vi "FF_compute2.vi"(0 "InitialCenter":dbl[](array[numeric]), 1 "CenPt":dbl[](array[numeric]), 2 "FrameNum":dbl, 7 "xyz_o":dbl[][](array[numeric]), 11 "New Center":dbl[](array[numeric]), 12 "Use FF":bool) -> (4 "P'":dbl[](array[numeric]), 5 "TraFF":dbl[](array[numeric]), 6 "curr Point":dbl[](array[numeric]), 8 "ForceAll":dbl[](array[numeric]), 10 "Closest Pt":dbl[](array[numeric]), 14 "InitalCenterOut":dbl[](array[numeric]), 15 "DesiredFM_FF":dbl[](array[numeric]))   [LabVIEW 2017]
uses:
  typeDef/AnkleTraj.ctl
  <vilib>/Analysis/_algsub.llb/Real Vector Norm.vi
  <vilib>/Analysis/baseanly.llb/Real Dot Product.vi
  <vilib>/Analysis/BLAS.llb/idamin - Min Element Index (DBL).vi
  <vilib>/Analysis/NI_AALBase.lvlib
  <vilib>/Analysis/NI_AALPro.lvlib
  <vilib>/Analysis/NI_AALBLAS.lvlib
panel:
  out "subarray 2":dbl[](array[numeric])
  out "subarray":dbl[](array[numeric])
  in  "Fz":dbl=20.0
  out "Desired FM_FF":dbl[](array[numeric])
  out "sqrt(x)":dbl
  out "P1 full size":i32[](array[numeric])
  out "P2 full":dbl[][](array[numeric])
  out "P1 full":dbl[][](array[numeric])
  out "CheckPlus":dbl[][](array[numeric])
  in  "AnkleTraj":T1
  out "OrderOfClosePt":i32
  in  "MxMyMz":dbl[](array[numeric])=[5.0, 5.0, 5.0, 4.0, 4.0, 4.0]
  in  "Enum":enum16{"Linear", "Bell"}(ring)=enum."Bell"
  out "ForceComp":dbl[](array[numeric])
  out "n_dir":dbl[](array[numeric])
  out "d_min":dbl
  out "ForceXYZ":dbl[](array[numeric])
  out "NormalVectorToClosestPt":dbl[](array[numeric])
  out "DistanceToClosestPt":dbl
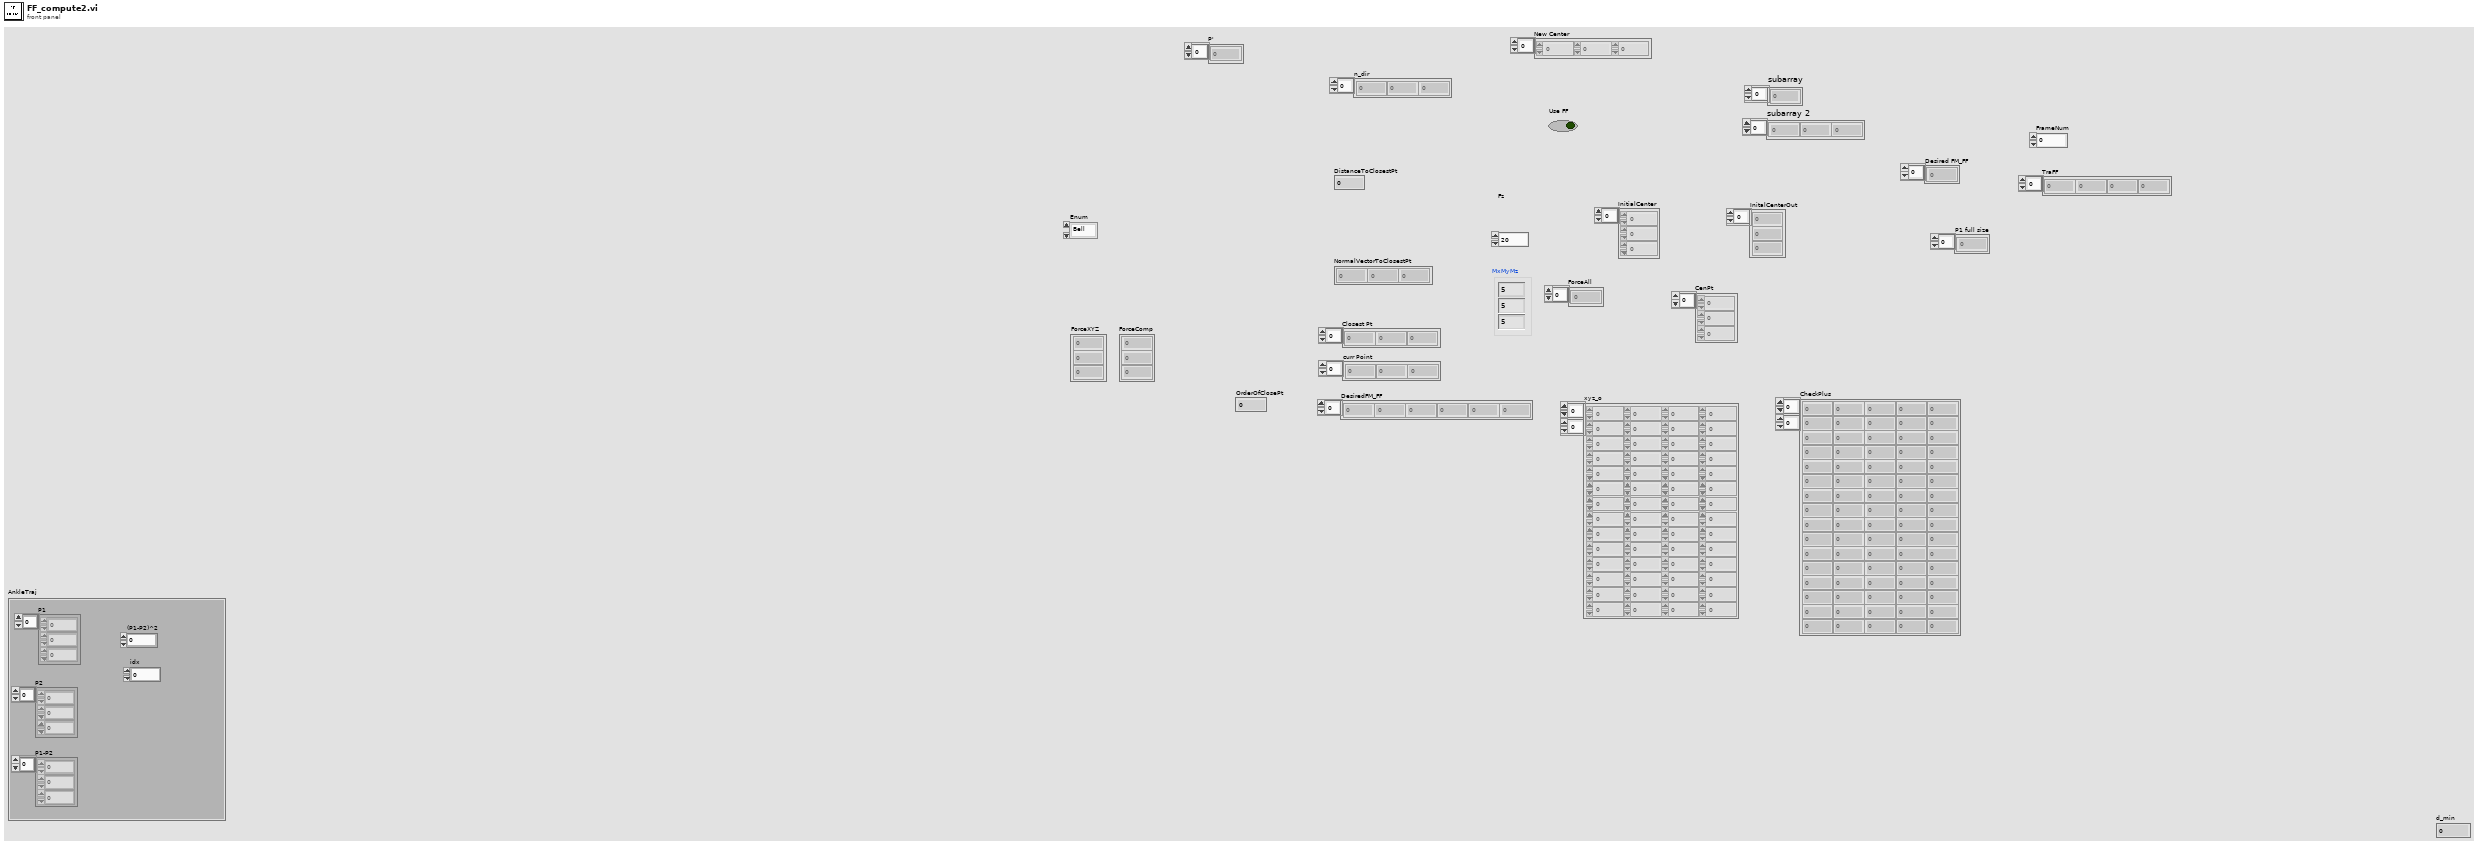
[diagram p1: front panel]
types:
  T1 = typedef "AnkleTraj.ctl" = cluster{"P1":dbl[], "P2":dbl[], "P1-P2":dbl[], "(P1-P2)^2":dbl, "idx":i32}
  T2 = cluster{"Kn":dbl, "Kt":dbl, "Kd_n":dbl, "Dn":dbl, "Dt":dbl, "Kd_t":dbl}
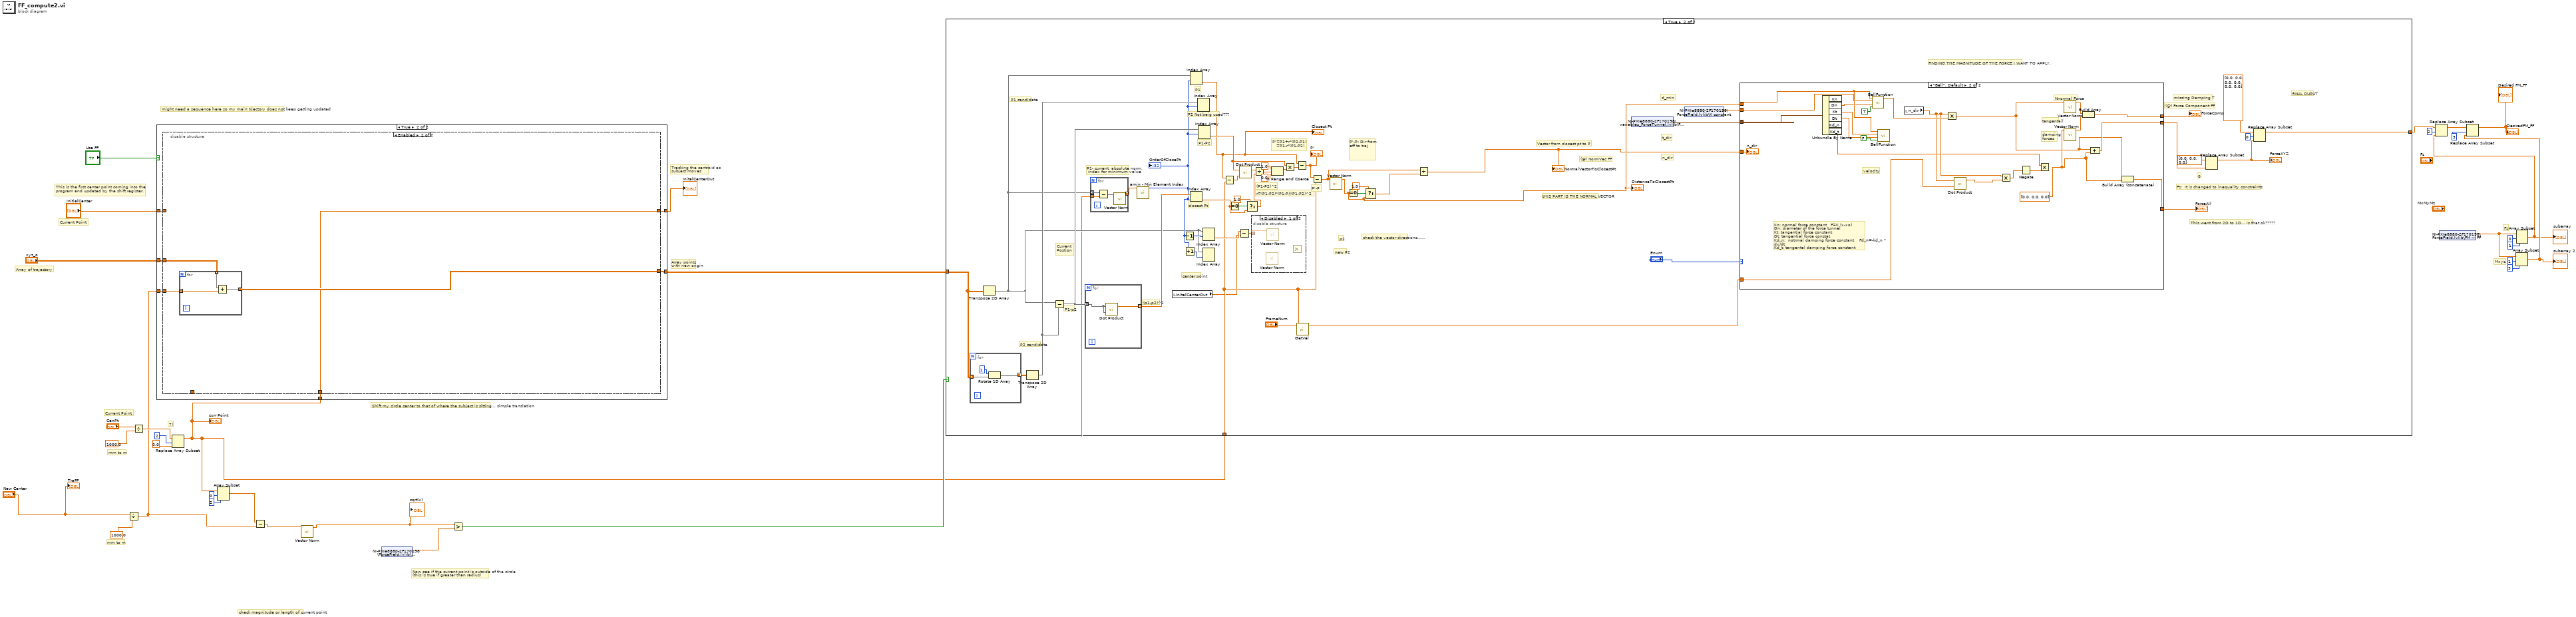
[diagram p0: block diagram]
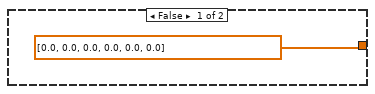
[diagram p2: hidden frame]
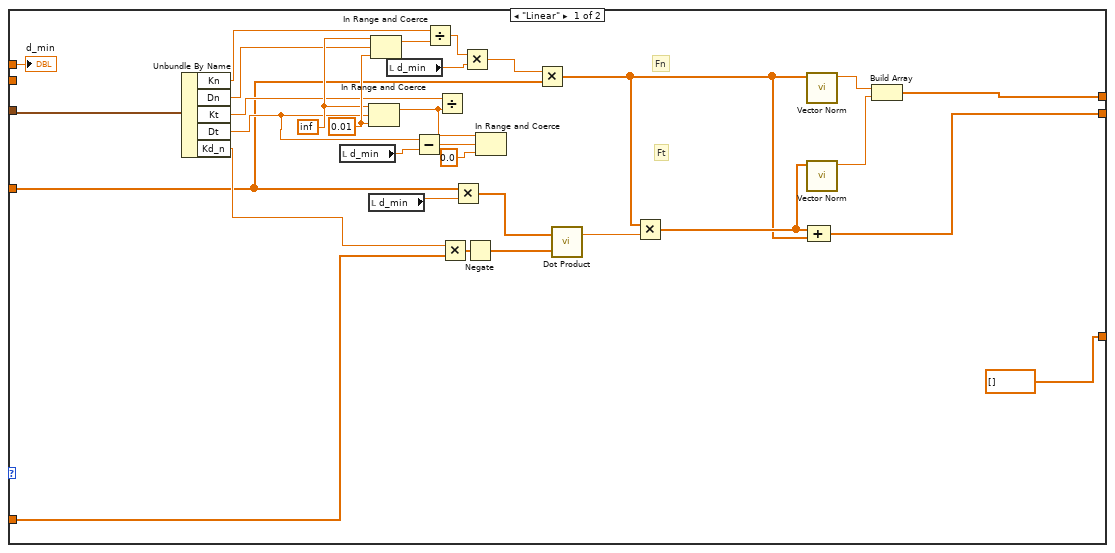
[diagram p4: hidden frame]
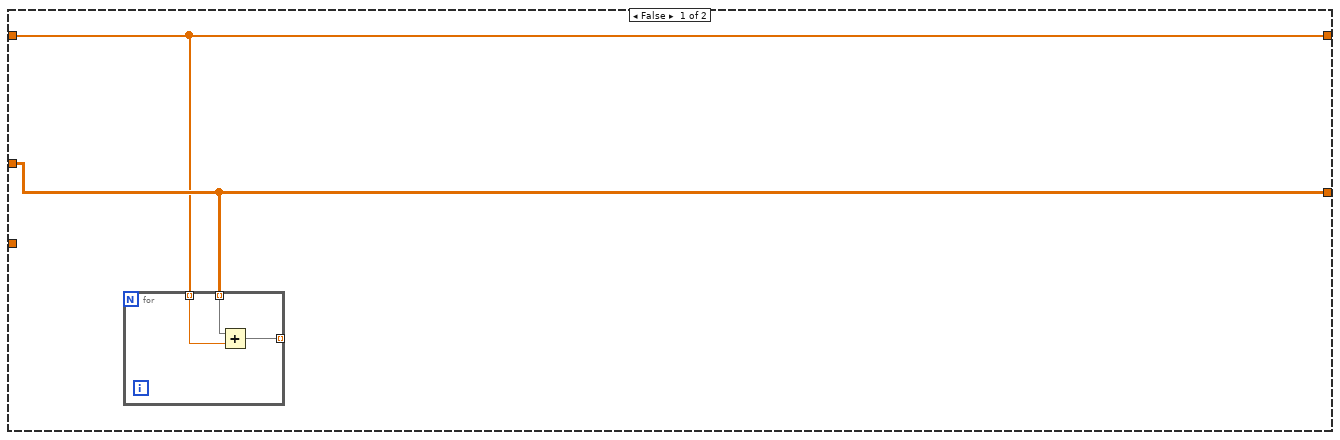
[diagram p5: hidden frame]
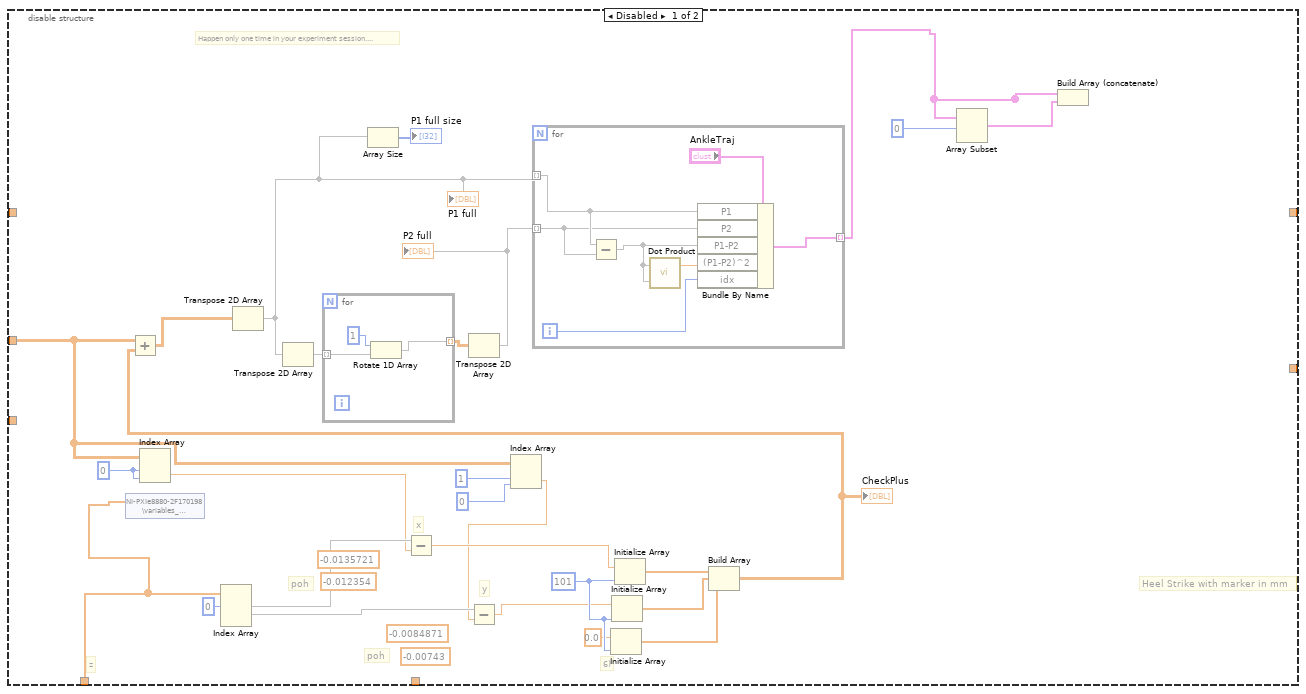
[diagram p6: hidden frame]
diagram:
  # "Current Point"
  # "Current Point"
  # "Fz"
  # "Mxyz"
  # "This is the first center point coming into the\nprogram and updated by the shift register."
  # "Now see if the current point is outside of the circle\n(this is true if greater than radius)"
  # "check magnitude or length of current point"
  # "mm to m"
  # "Tracking the centroid as \nsubject moves"
  # "might need a sequence here so my main trjectory does not keep getting updated"
  # "Array points \nwith new origin"
  # "Shift my circle center to that of where the subject is sitting... simple translation"
  # "mm to m"
  # "Array of trajectory"
  # "7)"
  n1 = Divide(x="New Center", y=1000.0) -> (x/y=w16:dbl[])
  n2 = Divide(x="CenPt", y=1000.0) -> (x/y=w28:dbl[])
  n3 = Replace Array Subset(array=w28, new element=0.0 ("new element/subarray"), index=2) -> (w15:dbl[])
  "curr Point" <- w15
  n4 = case shown="True" "Use FF" {
    tunnel: "xyz_o" -> [w35 w44]
    tunnel: [w35 w43] -> w26
    tunnel: "InitialCenter" -> [w34 w42]
    tunnel: [w34 w41] -> w24
    tunnel: w15 -> [_ w40]
    tunnel: w16 -> [_ w39]
    frame False {
      n5 = for {
        tunnel: w35 -> [w38] mode=indexing
        tunnel: [w37] -> _ mode=indexing
        tunnel: w34 -> [w36] mode=indexing
        n6 = Add(x=w38, y=w36) -> (x+y=w37:dbl[])
      }
    }
    frame True {
      n7 = disable-structure shown="Enabled" {
        disable-tunnel: _ -> [w51 _]
        disable-tunnel: w44 -> [w48 w86]
        disable-tunnel: [_ w85] -> w43
        disable-tunnel: w42 -> [_ _]
        disable-tunnel: [_ w84] -> w41
        disable-tunnel: w40 -> [_ w84]
        disable-tunnel: w39 -> [_ w83]
        frame Disabled {
          w50 = 0 ("index (row)")
          (unwired) -0.00743 ("x")
          (unwired) -0.012354 ("x")
          (unwired) -0.0084871 ("x")
          (unwired) -0.0135721 ("x")
          w65 = 101 ("dimension size")
          # "Happen only one time in your experiment session...."
          # "poh"
          # "poh"
          # "z"
          # "y"
          # "x"
          # "6)"
          # "Heel Strike with marker in mm"
          n8 = shared-variable "NI-PXIe8880-2F170198\\variables_ForceTunnel.lvlib\\Traj FF"(w51) -> ()  [unwired: 1 in, 1 out]
          n9 = Index Array(array=w48, index (row)=w50, index (col)=w50) -> (element=w49:dbl)
          n10 = Index Array(array=w51, index #1=0 ("index")) -> (element #1=w57, element #2=w59)  [unwired: 2 in, 1 out]
          n11 = Subtract(x=w57, y=w49) -> (x-y=w56:dbl)
          n12 = Index Array(array=w48, index (row)=1 ("disabled index (col)"), index (col)=0 ("index (row)")) -> (element=w47:dbl)
          n13 = Subtract(x=w59, y=w47) -> (x-y=w58:dbl)
          n14 = Initialize Array(0.0 ("element"), w65) -> (w63:dbl[])
          n15 = Initialize Array(w58, w65) -> (w64:dbl[])
          n16 = Initialize Array(w56, w65) -> (w55:dbl[])
          n17 = Build Array(w55, w64, w63) -> (w62:dbl[][])
          "CheckPlus" <- w62
          n18 = Add(x=w48, y=w62) -> (x+y=w61:dbl[][])
          n19 = Transpose 2D Array(2D array=w61) -> (transposed array=w54:dbl[][])
          "P1 full" <- w54
          n20 = Transpose 2D Array(2D array=w54) -> (transposed array=w69:dbl[][])
          n21 = for {
            tunnel: w69 -> [w82] mode=indexing
            tunnel: [w81] -> w68 mode=indexing
            n22 = Rotate 1D Array(1:w82, 2:1 ("n")) -> (0:w81:dbl[])
          }
          n23 = Array Size(array=w54) -> (size(s)=→"P1 full size":i32[])
          n24 = Transpose 2D Array(2D array=w68) -> (transposed array=w52:dbl[][])
          "P2 full" <- w52
          n25 = for {
            tunnel: w54 -> [w78] mode=indexing
            tunnel: w52 -> [w77] mode=indexing
            tunnel: [w74] -> w67 mode=indexing
            i -> [w73]
            n26 = Subtract(x=w78, y=w77) -> (x-y=w75:dbl[])
            n27 = call-poly <vilib>:"Dot Product.vi"("Y Vector"=w75, "X Vector"=w75) -> ("X * Y"=w76:dbl)  [unwired: 1 out]
            n28 = Bundle By Name(cluster="AnkleTraj", "P1"=w78, "P2"=w77, "P1-P2"=w75, "(P1-P2)^2"=w76, "idx"=w73) -> (w74:T1)
          }
          n29 = Array Subset(array=w67, index=0) -> (w72:T1[])  [unwired: 1 in]
          n30 = Build Array (concatenate)(w67, w72) -> (w71:T1[])
        }
        frame Enabled {
          n31 = for {
            tunnel: w86 -> [w89] mode=indexing
            tunnel: [w88] -> w85 mode=indexing
            tunnel: w83 -> [w87] mode=indexing
            n32 = Add(x=w89, y=w87) -> (x+y=w88:dbl[])
          }
        }
      }
    }
  }
  "InitalCenterOut" <- w24
  n33 = Array Subset(array=w15, index=0, length=2) -> (w12:dbl[])
  n34 = Subtract(x=w12, y=w16) -> (x-y=w11:dbl[])
  n35 = call-poly <vilib>:"Vector Norm.vi"("Input Vector"=w11) -> ("norm"=w10:dbl)  [unwired: 9 in, 1 out]
  "sqrt(x)" <- w10
  n36 = shared-variable "NI-PXIe8880-2F170198\\ForceField.lvlib\\Radius"() -> (w1:dbl)  [unwired: 1 in, 1 out]
  n37 = Greater?(x=w10, y=w1) -> (0:w22:bool)
  n38 = case shown="True" w22 {
    tunnel: [dbl[] [0.0, 0.0, 0.0, 0.0, 0.0, 0.0] w92] -> w19
    tunnel: w26 -> [_ w96]
    tunnel: w15 -> [_ w94]
    frame False {
    }
    frame True {
      # "P2 Not beig used???"
      # "This went from 2D to 1D... is that ok?????"
      # "P1- current, absolute norm,\n index for minimum value"
      # "check the vector directions......"
      # "p1"
      # "new P2"
      # "center point"
      # "(p1-p2)^2"
      # "P1-p2"
      # "P1 candidate"
      # "P2 candidate"
      # "fINAL OUPUT"
      # "tHIS PART IS THE NORMAL VECTOR"
      # "FINDING THE MAGNITUDE OF THE FORCE I WANT TO APPLY."
      # "missing Damping T"
      # "0"
      # "Fz:  It is changed to inequality constraints"
      # "(@) Force Component FF"
      # "(@) NormVec FF"
      # "(P1-P2)^2"
      # "closest Pt"
      # "P1-P2"
      # "P1"
      # "P'-P"
      # "P'-P: Dir from eff to traj"
      # "r=(P1-P2)*(P1-P)/(P1-P2)^2"
      # "P'=P1+r*(P2-P1)\n   =P1-r*(P1-P2)"
      # "Current \nPostion"
      # "t_dir"
      # "n_dir"
      # "d_min"
      # "Vector from closest pt to P"
      n39 = for {
        tunnel: w96 -> [w147] mode=indexing
        tunnel: [w146] -> w107 mode=indexing
        n40 = Rotate 1D Array(1:w147, 2:1 ("n")) -> (0:w146:dbl[])
      }
      n41 = Transpose 2D Array(2D array=w96) -> (transposed array=w95:dbl[][])
      n42 = Transpose 2D Array(2D array=w107) -> (transposed array=w98:dbl[][])
      n43 = Subtract(x=w95, y=w98) -> (x-y=w102:dbl[][])
      n44 = for {
        tunnel: w102 -> [w144] mode=indexing
        tunnel: [w143] -> w101 mode=indexing
        n45 = call-poly <vilib>:"Dot Product.vi"("Y Vector"=w144, "X Vector"=w144) -> ("X * Y"=w143:dbl)  [unwired: 1 out]
      }
      n46 = for {
        tunnel: w94 -> [w142] mode=indexing
        tunnel: w95 -> [w141] mode=indexing
        tunnel: [w139] -> w100 mode=indexing
        n47 = Subtract(x=w141, y=w142) -> (x-y=w140:dbl[])
        n48 = call-poly <vilib>:"Vector Norm.vi"("Input Vector"=w140) -> ("norm"=w139:dbl)  [unwired: 9 in, 1 out]
      }
      n49 = call-poly <vilib>:"amin - Min Element Index.vi"("x"=w100) -> ("idamin"=w97:i32)  [unwired: 9 in, 1 out]
      "OrderOfClosePt" <- w97
      n50 = local read "InitalCenterOut"() -> (w93:dbl[])
      n51 = Decrement(x=w97) -> (x-1=w106:i32)
      n52 = Increment(x=w97) -> (x+1=w105:i32)
      n53 = Index Array(array=w95, index (row)=w97) -> (element=w116:dbl[])  [unwired: 1 in]
      "Closest Pt" <- w116
      n54 = Index Array(array=w101, index=w97) -> (element=w110:dbl)
      n55 = Index Array(array=w98, index (row)=w97) -> ()  [unwired: 1 in, 1 out]
      n56 = Index Array(array=w102, index (row)=w97) -> (element=w123:dbl[])  [unwired: 1 in]
      n57 = Index Array(array=w95, index (row)=w106) -> (element=w104:dbl[])  [unwired: 1 in]
      n58 = Index Array(array=w95, index (row)=w105) -> ()  [unwired: 1 in, 1 out]
      n59 = Subtract(x=w116, y=w94) -> (x-y=w130:dbl[])
      n60 = Equal To 0?(x=w110) -> (x = 0?=w112:bool)
      n61 = Subtract(x=w104, y=w93) -> (x-y=w103:dbl[])
      n62 = call-poly <vilib>:"Dot Product.vi"("Y Vector"=w130, "X Vector"=w123) -> ("X * Y"=w129:dbl)  [unwired: 1 out]
      n63 = Select(t=1.0, s=w112, f=w110) -> (s? t:f=w109:dbl)
      n64 = disable-structure shown="Disabled" {
        disable-tunnel: w103 -> [w138 _]
        frame Disabled {
          n65 = call-poly <vilib>:"Vector Norm.vi"() -> ()  [unwired: 10 in, 2 out]
          n66 = call-poly <vilib>:"Vector Norm.vi"("Input Vector"=w138) -> ()  [unwired: 9 in, 2 out]
          n67 = Greater?() -> ()  [unwired: 2 in, 1 out]
        }
        frame Enabled {
        }
      }
      n68 = Divide(x=w129, y=w109) -> (x/y=w128:dbl)
      n69 = In Range and Coerce(upper limit=1.0, x=w128, lower limit=0.0) -> (coerced(x)=w125:dbl)  [unwired: 1 out]
      n70 = Multiply(x=w123, y=w125) -> (x*y=w124:dbl[])
      n71 = Subtract(x=w116, y=w124) -> (x-y=w121:dbl[])
      "P'" <- w121
      n72 = call "GetVel.vi"("Position"=w94, "FrameNum"="FrameNum") -> ("Velocity"=w118:dbl[])  [unwired: 9 in]
      n73 = Subtract(x=w121, y=w94) -> (x-y=w122:dbl[])
      n74 = call-poly <vilib>:"Vector Norm.vi"("Input Vector"=w122) -> ("norm"=w108:dbl)  [unwired: 9 in, 1 out]
      "DistanceToClosestPt" <- w108
      n75 = Equal To 0?(x=w108) -> (x = 0?=w115:bool)
      n76 = Select(t=1.0, s=w115, f=w108) -> (s? t:f=w113:dbl)
      n77 = Divide(x=w122, y=w113) -> (x/y=w120:dbl[])
      "NormalVectorToClosestPt" <- w120
      n78 = shared-variable "NI-PXIe8880-2F170198\\variables_ForceTunnel.lvlib\\FF Constant"() -> (w117:T2)  [unwired: 1 in, 1 out]
      n79 = shared-variable "NI-PXIe8880-2F170198\\ForceField.lvlib\\K constant"() -> (w91:dbl)  [unwired: 1 in, 1 out]
      n80 = case shown="\"Bell\", Default" "Enum" {
        tunnel: [w178 w198] -> w131
        tunnel: [w160 w201] -> w135
        tunnel: w118 -> [w177 w184]
        tunnel: w117 -> [w159 w197]
        tunnel: w108 -> [w152 w191]
        tunnel: w120 -> [w153 w192]
        tunnel: [dbl[] [] w182] -> w99
        tunnel: w91 -> [_ w180]
        frame "Linear" {
          w165 = inf
          w166 = 0.01 ("upper limit")
          # "Ft"
          # "Fn"
          n81 = Unbundle By Name(w159) -> ("Kn"=w158:dbl, "Dn"=w157:dbl, "Kt"=w156:dbl, "Dt"=w155:dbl, "Kd_n"=w154:dbl)
          n82 = local read "d_min"() -> (w150:dbl)
          n83 = In Range and Coerce(upper limit=w165, x=w155, lower limit=w166) -> (coerced(x)=w167:dbl)  [unwired: 1 out]
          n84 = local read "d_min"() -> (w149:dbl)
          n85 = In Range and Coerce(upper limit=w165, x=w157, lower limit=w166) -> (coerced(x)=w168:dbl)  [unwired: 1 out]
          n86 = local read "d_min"() -> (w151:dbl)
          n87 = Subtract(x=w155, y=w150) -> (x-y=w170:dbl)
          n88 = Divide(x=w158, y=w168) -> (x/y=w164:dbl)
          n89 = Divide(x=w156, y=w167) -> ()  [unwired: 1 out]
          n90 = Multiply ("Multiply.vi")(x=w154, y=w177) -> (x*y=w174:dbl[])
          n91 = Multiply(x=w153, y=w149) -> (x*y=w173:dbl[])
          n92 = Multiply(x=w164, y=w151) -> (x*y=w163:dbl)
          n93 = Negate(x=w174) -> (-x=w172:dbl[])
          n94 = In Range and Coerce(upper limit=w167, x=w170, lower limit=0.0) -> ()  [unwired: 2 out]
          n95 = Multiply(x=w163, y=w153) -> (x*y=w161:dbl[])
          n96 = call-poly <vilib>:"Dot Product.vi"("Y Vector"=w172, "X Vector"=w173) -> ("X * Y"=w171:dbl)  [unwired: 1 out]
          n97 = Multiply(x=w161, y=w171) -> (x*y=w162:dbl[])
          n98 = call-poly <vilib>:"Vector Norm.vi"("Input Vector"=w161) -> ("norm"=w175:dbl)  [unwired: 9 in, 1 out]
          n99 = call-poly <vilib>:"Vector Norm.vi"("Input Vector"=w162) -> ("norm"=w176:dbl)  [unwired: 9 in, 1 out]
          n100 = Compound Arithmetic op=ADD(w162, w161) -> (w160:dbl[])
          n101 = Build Array(w175, w176) -> (w178:dbl[])
          "d_min" <- w152
        }
        frame "Bell", Default {
          w181 = dbl[] [0.0, 0.0, 0.0] ("x*y")
          # "damping \nforces"
          # "tangentail"
          # "Nnormal Force"
          # "Kn: normal force constant   F=K (x-xo)\nDn: diameter of the force tunnel\nKt: tangential force constant\nDt: tangential force constat\nKd_n:  notrmal damping force constant    Fd_n=-kd_n * dx/dt\nKd_t: tangental damping force constant"
          # "velocity"
          n102 = Unbundle By Name(w197) -> ("Dn"=w179:dbl, "Kt"=w193:dbl, "Dt"=w194:dbl, "Kd_n"=w186:dbl)  [unwired: 2 out]
          n103 = call "BellFunction.vi"("Invert"=TRUE, "(r)adius"=w179, "(A)mplitude"=w180, "x"=w191) -> ("y"=w190:dbl)  [unwired: 2 in]
          n104 = call "BellFunction.vi"("Invert"=FALSE, "(r)adius"=w194, "(A)mplitude"=w193, "x"=w191) -> ()  [unwired: 2 in, 1 out]
          n105 = local read "n_dir"() -> (w188:dbl[])
          n106 = Multiply(x=w188, y=w190) -> (x*y=w183:dbl[])
          n107 = call-poly <vilib>:"Dot Product.vi"("Y Vector"=w184, "X Vector"=w188) -> ("X * Y"=w189:dbl)  [unwired: 1 out]
          n108 = Multiply(x=w188, y=w189) -> (x*y=w187:dbl[])
          n109 = Negate(x=w187) -> (-x=w185:dbl[])
          n110 = Multiply(x=w186, y=w185) -> ()  [unwired: 1 out]
          n111 = call-poly <vilib>:"Vector Norm.vi"("Input Vector"=w183) -> ("norm"=w200:dbl)  [unwired: 9 in, 1 out]
          n112 = call-poly <vilib>:"Vector Norm.vi"("Input Vector"=w181) -> ("norm"=w199:dbl)  [unwired: 9 in, 1 out]
          n113 = Build Array(w200, w199) -> (w198:dbl[])
          n114 = Compound Arithmetic op=ADD(w183, w181) -> (w201:dbl[])
          n115 = Build Array (concatenate)(w183, w181) -> (w182:dbl[])
          "n_dir" <- w192
        }
      }
      "ForceComp" <- w131
      "ForceAll" <- w99
      n116 = Replace Array Subset(array=dbl[] [0.0, 0.0, 0.0], new element=w135) -> (w132:dbl[])  [unwired: 1 in]
      "ForceXYZ" <- w132
      n117 = Replace Array Subset(array=dbl[] [0.0, 0.0, 0.0, 0.0, 0.0, 0.0] ("element"), new element=w132, index=0) -> (w92:dbl[])
    }
  }
  n118 = shared-variable "NI-PXIe8880-2F170198\\ForceField.lvlib\\FM --- FF"() -> (w8:dbl[])  [unwired: 1 in, 1 out]
  n119 = Array Subset(array=w8, index=1, length=3) -> (w3:dbl[])
  "subarray 2" <- w3
  n120 = Array Subset(array=w8, index=0, length=1) -> (w2:dbl[])
  "subarray" <- w2
  n121 = Replace Array Subset(array=w19, new element=w2, index=2) -> (w18:dbl[])
  n122 = Replace Array Subset(array=w18, new element=w3, index=3) -> (→"DesiredFM_FF" →"Desired FM_FF":dbl[])
  "TraFF" <- "New Center"
